vi "FTW-Actor-Destroy.vi"(0 "FTW Actor Instance":refnum<class "FTW-ActorInstance.lvclass">, 5 "Force Destroy?":bool=TRUE, 11 "error in":errorcluster) -> (15 "error out":errorcluster)   [LabVIEW 2015, in "FTW-ActorInstance.lvclass"]
uses:
  FTW-ActorInstance.lvclass
  FTW-Actor-FrameworkEvent.ctl
  <vilib>/event_ctls.llb/usereventprio.ctl
  FTW-ActorInstance.lvclass/FTW-ActorInstance.ctl
  EventLogger/FTW-Logger.lvclass
  JobSequencer/FTW-JobSequencer.lvclass
  Reply/FTW-Reply.lvclass
panel:
  # "Inputs"
  # "Outputs"
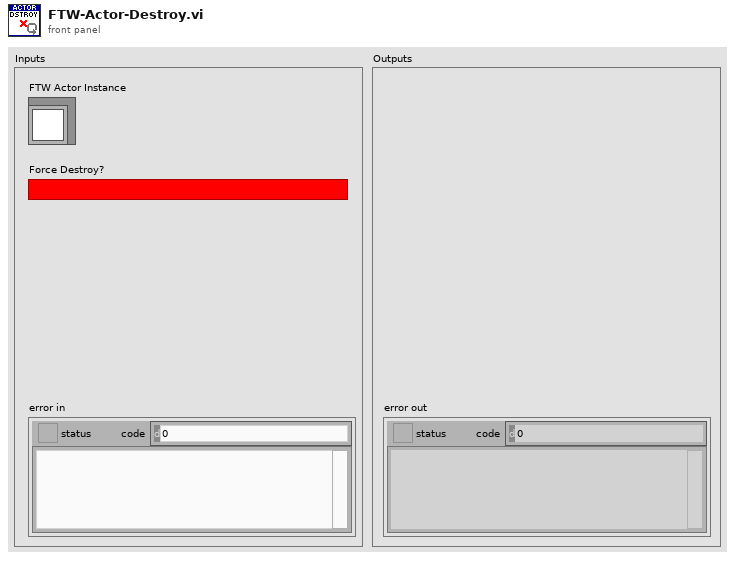
[diagram p1: front panel]
types:
  T1 = typedef "usereventprio.ctl" = enum32{"high priority", "normal priority"}
  T2 = typedef "FTW-ActorInstance.lvclass/FTW-Actor-FrameworkEvent.ctl" = enum16{"Instance Initializing", "Instance Constructed", "Instance Initialized", "Instance Job", "Instance Handle Request", "Instance Shutting Down", "Instance Destroyed"}
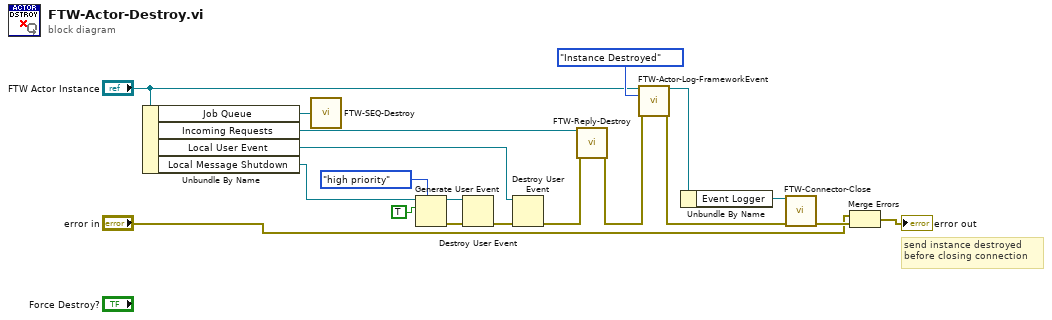
[diagram p0: block diagram]
diagram:
  # "send instance destroyed\nbefore closing connection"
  n1 = Unbundle By Name("FTW Actor Instance") -> ("Job Queue"=w19:refnum<class "FTW-JobSequencer.lvclass">, "Incoming Requests"=w18:refnum<class "FTW-Reply.lvclass">, "Local User Event"=w9:refnum<user-event>, "Local Message Shutdown"=w6:refnum<user-event>)
  n2 = call "FTW-SEQ-Destroy.vi"("FTW Job Sequencer"=w19) -> ()  [unwired: 1 in]
  n3 = Generate User Event(priority (normal)=usereventprio."high priority", user event=w6, event data cluster=TRUE ("event data")) -> (user event out=w5:refnum<user-event>, error out=w7:errorcluster)  [unwired: 1 in]
  n4 = Destroy User Event(user event=w5, error in=w7) -> (error out=w8:errorcluster)
  n5 = Destroy User Event(user event=w9, error in=w8) -> (error out=w10:errorcluster)
  n6 = call "FTW-Reply-Destroy.vi"("FTW-Router In"=w18, "error in"=w10) -> ("error out"=w11:errorcluster)  [unwired: 13 in]
  n7 = call "FTW-Actor-Log-FrameworkEvent.vi"("FTW Actor Instance"="FTW Actor Instance", "Framework Event"=FTW-Actor-FrameworkEvent."Instance Destroyed", "error in"=w11) -> ("FTW Actor Instance out"=w13:refnum<class "FTW-ActorInstance.lvclass">, "error out"=w14:errorcluster)  [unwired: 11 in]
  n8 = Unbundle By Name(w13) -> ("Event Logger"=w12:refnum<class "FTW-Logger.lvclass">)
  n9 = call-dynamic "FTW-Connector-Close.vi"("FTW Actor Connector"=w12, "error in"=w14) -> ("error out"=w17:errorcluster)  [unwired: 13 in]
  n10 = Merge Errors("error in", w17) -> (→"error out":errorcluster)
